vi "read_environment (SubVI).vi"(10 "Read pressures?":bool, 11 "Read temps?":bool) -> (3 "environ cluster":cluster{dbl[], dbl[]})   [LabVIEW 2022 SP3]
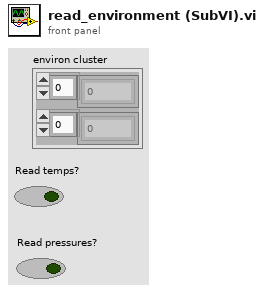
[diagram p1: front panel]
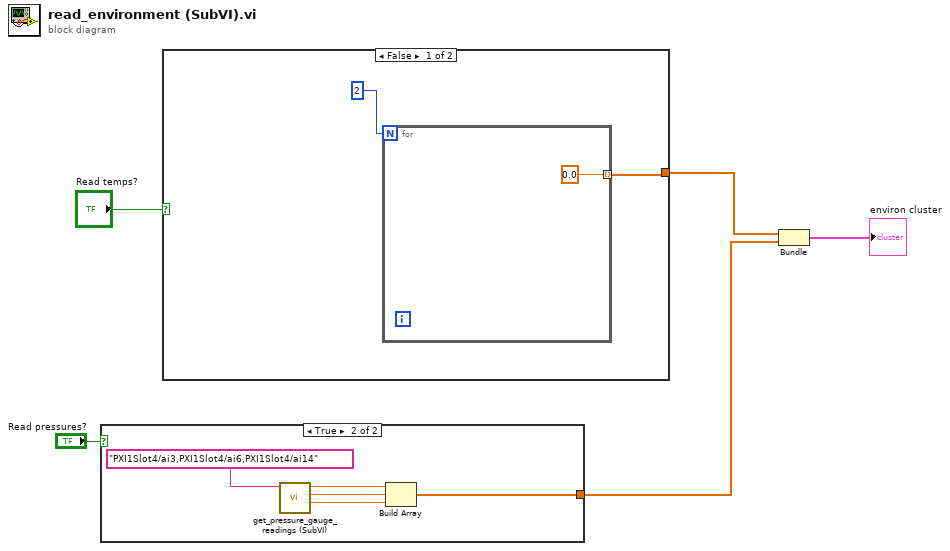
[diagram p0: block diagram]
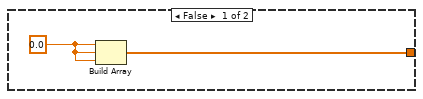
[diagram p2: hidden frame]
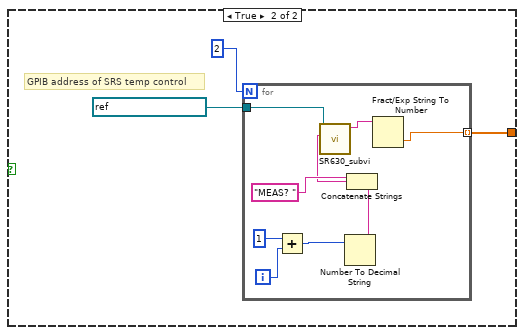
[diagram p3: hidden frame]
diagram:
  n1 = case shown="True" "Read pressures?" {
    tunnel: [w6 w12] -> w1
    frame False {
      w7 = 0.0 ("element")
      n2 = Build Array(w7, w7, w7) -> (w6:dbl[])
    }
    frame True {
      n3 = call "get_pressure_gauge_readings (SubVI).vi"("pressure_gauge_monitors"=tag "PXI1Slot4/ai3,PXI1Slot4/ai6,PXI1Slot4/ai14" ("Channel 1")) -> ("baratron"=w8:dbl, "1torr_baratron"=w9:dbl, "pirani"=w10:dbl)  [unwired: 7 in, 1 out]
      n4 = Build Array(w10, w9, w8) -> (w12:dbl[])
    }
  }
  n5 = case shown="False" "Read temps?" {
    tunnel: [w13 w16] -> w4
    frame False {
      n6 = for {
        N: 2 ("dimension size") -> [_]
        tunnel: [0.0] -> w13 mode=indexing
      }
    }
    frame True {
      # "GPIB address of SRS temp control"
      n7 = for {
        N: 2 ("dimension size") -> [_]
        tunnel: refnum<visa-resource-name> "GPIB0::19::INSTR" ("VISA Refnum in") -> [w27]
        tunnel: [w25] -> w16 mode=indexing
        i -> [w24]
        n8 = Add(x=1, y=w24) -> (x+y=w22:i32)
        n9 = Number To Decimal String(number=w22) -> (decimal integer string=w21:string)  [unwired: 1 in]
        n10 = Concatenate Strings("MEAS? " ("Write Buffer"), w21) -> (w19:string)
        n11 = call "SR630_subvi.vi"("Write Buffer"=w19, "VISA Refnum in"=w27) -> ("read buffer"=w26:string)  [unwired: 9 in]
        n12 = Fract/Exp String To Number(string=w26) -> (number=w25:dbl)  [unwired: 3 in, 1 out]
      }
    }
  }
  n13 = Bundle(w4, w1) -> (→"environ cluster":cluster{dbl[], dbl[]})  [unwired: 1 in]
